vi "U8.vi"(8 "Error In":errorcluster) -> (0 "Error Out":errorcluster)   [LabVIEW 2018, in "Tests.lvlib" / "To Msgpack.lvlib"]
uses:
  To Msgpack.lvlib
  <vilib>/addons/_JKI Toolkits/Caraya/classes/Test/Test.lvclass
  src/LabPack/Toolkit.lvlib
  <vilib>/addons/_JKI Toolkits/Caraya/classes/Assert/Assert.lvclass
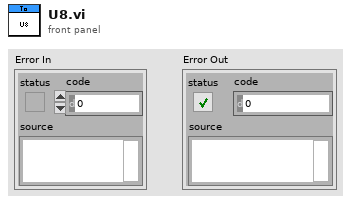
[diagram p1: front panel]
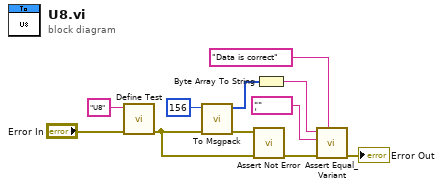
[diagram p0: block diagram]
diagram:
  n1 = call <vilib>:"Define Test.vi"("error in (no error)"="Error In", "Label (VI Title)"="U8") -> ("error out"=w7:errorcluster)  [unwired: 9 in]
  n2 = call "To Msgpack.vi"("Error In"=w7, "Anything"=u8 156) -> ("Error Out"=w8:errorcluster, "Msgpack Data"=w5:u8[])  [unwired: 8 in]
  n3 = call <vilib>:"Assert Not Error.vi"("error in (no error)"=w7, "Not Error?"=w8) -> ("error out"=w9:errorcluster)  [unwired: 9 in]
  n4 = Byte Array To String(unsigned byte array=w5) -> (string=w4:string)
  n5 = call <vilib>:"Assert Equal_Variant.vi"("Label"="Data is correct", "error in (no error)"=w9, "Y"="̜" ("string"), "X"=w4) -> ("error out"=→"Error Out":errorcluster)  [unwired: 7 in]
